vi "Facade.vi"(0 "Data In":T25={"Waveform"={"Type"=enum."Tone", "Tone"={"Frequency (kHz)"=0.0, "Last Freq"=0.0, "Last Phase"=0.0}, "Pulse Train"={"Pulse width (us)"=0.0, "Pulse rate (Hz)"=0.0, "Gap (ms)"=0.0, "Polarity"=enum."POS", "PT State"={"Template"=[], "Nperiod"=0, "Index"=0, "Pulse Rate (Hz)"=0.0, "Phase (cycles)"=0.0, "Noff"=0}, "Asynch"=FALSE}, "Noise"={"InvFilt"=FALSE, "Noise"=[], "CurPt"=0, "Aweight"=FALSE, "Seed"=0, "afile"=path ""}, "File"={"Filename"=path "", "Signal"=[], "Channel"=0, "stream"=FALSE, "offset"=0, "nreps"=0, "loops"=0, "Randomize"=FALSE, "order"=[], "Seed"=0, "Tokens"=0}, "FMSweep"={"Rate (oct/s)"=0.0, "Fmin (Hz)"=0.0, "Fmax (Hz)"=0.0, "Ramp (ms)"=0.0, "Linear"=FALSE}, "Chirp Train"={"Params"={"Fmin (kHz)"=4.0, "Fmax (kHz)"=64.0, "Compensate"=FALSE, "Duration (ms)"=2.0}, "Data"={"WF"=[]}}, "Complex Tone"={"Params"={"F0 (Hz)"=0.0, "Band"={"Flow (Hz)"=0.0, "Fhigh (Hz)"=0.0}, "Phase"=enum."Cosine", "Min F0 (Hz)"=0.0, "Max F0 (Hz)"=0.0, "ContinRandPhase"=FALSE, "Max peak factor"=inf, "Max mod depth"=2.0, "MinHarmNum"=0, "MaxHarmNum"=0, "Level Mode"=enum."per component", "% jitter"=0.0}, "Data"={"Ncomp"=0, "MinHarm"=0, "Phase"=[], "Amplitude"=[], "Npts/frame"=0, "Last F0"=0.0, "Fmin"=0.0, "Fmax"=0.0, "Lslope"=0.0, "randphase"=FALSE, "overall rms"=FALSE, "fmult"=[], "jittered"=FALSE}}, "Moving Ripple"={"Params"={"Fmin"=0.0, "Fmax"=0.0, "Density"=0.0, "Velocity"=0.0, "Depth"=0.0, "Phase"=0.0, "Comp/oct"=0}, "Data"={"Freq"=[], "A"=[], "phase"=[], "Phase"=0.0}}}, "Filter"={"CF (kHz)"=0.0, "BW (kHz)"=0.0, "IIR Filter Cluster"={"filter structure"=enum."IIR 2nd Order", "Reverse Coefficients"=[], "Forward Coefficients"=[]}, "Final Filter State"=[], "Scale Factor"=0.0, "Final Filter State 2"=[], "Quadrature"=FALSE, "Type"=enum."Lowpass"}, "Gate"={"Active"=FALSE, "Delay (ms)"=0.0, "Width (ms)"=50.0, "Ramp (ms)"=5.0}, "Level"={"Level"=0.0, "Units"=enum."dB atten", "Max"=0.0, "Multiplier"=0.0, "Cal File"=path "", "Cal"={"Freq (Hz)"=[], "Mag (dB SPL)"=[], "Phase (deg)"=[]}}} {"Filter"."IIR Filter Cluster"."Forward Coefficients" format="%.4f"; "Filter"."IIR Filter Cluster"."Reverse Coefficients" format="%.4f"}, 2 "Display State In":T23, 3 "Container State":T24) -> (6 "Data Out":T25={"Waveform"={"Type"=enum."Tone", "Tone"={"Frequency (kHz)"=0.0, "Last Freq"=0.0, "Last Phase"=0.0}, "Pulse Train"={"Pulse width (us)"=0.0, "Pulse rate (Hz)"=0.0, "Gap (ms)"=0.0, "Polarity"=enum."POS", "PT State"={"Template"=[], "Nperiod"=0, "Index"=0, "Pulse Rate (Hz)"=0.0, "Phase (cycles)"=0.0, "Noff"=0}, "Asynch"=FALSE}, "Noise"={"InvFilt"=FALSE, "Noise"=[], "CurPt"=0, "Aweight"=FALSE, "Seed"=0, "afile"=path ""}, "File"={"Filename"=path "", "Signal"=[], "Channel"=0, "stream"=FALSE, "offset"=0, "nreps"=0, "loops"=0, "Randomize"=FALSE, "order"=[], "Seed"=0, "Tokens"=0}, "FMSweep"={"Rate (oct/s)"=0.0, "Fmin (Hz)"=0.0, "Fmax (Hz)"=0.0, "Ramp (ms)"=0.0, "Linear"=FALSE}, "Chirp Train"={"Params"={"Fmin (kHz)"=4.0, "Fmax (kHz)"=64.0, "Compensate"=FALSE, "Duration (ms)"=2.0}, "Data"={"WF"=[]}}, "Complex Tone"={"Params"={"F0 (Hz)"=0.0, "Band"={"Flow (Hz)"=0.0, "Fhigh (Hz)"=0.0}, "Phase"=enum."Cosine", "Min F0 (Hz)"=0.0, "Max F0 (Hz)"=0.0, "ContinRandPhase"=FALSE, "Max peak factor"=inf, "Max mod depth"=2.0, "MinHarmNum"=0, "MaxHarmNum"=0, "Level Mode"=enum."per component", "% jitter"=0.0}, "Data"={"Ncomp"=0, "MinHarm"=0, "Phase"=[], "Amplitude"=[], "Npts/frame"=0, "Last F0"=0.0, "Fmin"=0.0, "Fmax"=0.0, "Lslope"=0.0, "randphase"=FALSE, "overall rms"=FALSE, "fmult"=[], "jittered"=FALSE}}, "Moving Ripple"={"Params"={"Fmin"=0.0, "Fmax"=0.0, "Density"=0.0, "Velocity"=0.0, "Depth"=0.0, "Phase"=0.0, "Comp/oct"=0}, "Data"={"Freq"=[], "A"=[], "phase"=[], "Phase"=0.0}}}, "Filter"={"CF (kHz)"=0.0, "BW (kHz)"=0.0, "IIR Filter Cluster"={"filter structure"=enum."IIR 2nd Order", "Reverse Coefficients"=[], "Forward Coefficients"=[]}, "Final Filter State"=[], "Scale Factor"=0.0, "Final Filter State 2"=[], "Quadrature"=FALSE, "Type"=enum."Lowpass"}, "Gate"={"Active"=FALSE, "Delay (ms)"=0.0, "Width (ms)"=50.0, "Ramp (ms)"=5.0}, "Level"={"Level"=0.0, "Units"=enum."dB atten", "Max"=0.0, "Multiplier"=0.0, "Cal File"=path "", "Cal"={"Freq (Hz)"=[], "Mag (dB SPL)"=[], "Phase (deg)"=[]}}} {"Filter"."IIR Filter Cluster"."Forward Coefficients" format="%.4f"; "Filter"."IIR Filter Cluster"."Reverse Coefficients" format="%.4f"}, 7 "Display State Out":T23, 8 "Action":T22)   [LabVIEW 2020, in "Stimulus Channel.xctl"]
uses:
  Stimulus Channel.xctl
  Stimulus Channel Data.ctl
  Waveform XCtl/Waveform Data.ctl
  Waveform XCtl/Waveform Enum.ctl
  Waveform VIs/Tone VIs/Tone Params.ctl
  Waveform VIs/Pulse Train VIs/Pulse Train Params.ctl
  Waveform VIs/Pulse Train VIs/Pulse Polarity.ctl
  Waveform VIs/Pulse Train VIs/PT-Continuous State.ctl
  Waveform VIs/Noise VIs/Noise Params.ctl
  Waveform VIs/File VIs/StimFile-Params.ctl
  Waveform VIs/FM Sweep VIs/FM Sweep Params.ctl
  Waveform VIs/Chirp Train VIs/Chirp Train.ctl
  Waveform VIs/Chirp Train VIs/Chirp Train Params.ctl
  Waveform VIs/Complex Tone VIs/CT-Params.ctl
  Waveform VIs/Complex Tone VIs/CT-Phase Enum.ctl
  Waveform VIs/Complex Tone VIs/CT-Runtime Data.ctl
  Waveform VIs/Moving Ripple VIs/Moving Ripple.ctl
  Waveform VIs/Moving Ripple VIs/Moving Ripple.Params.ctl
  Waveform VIs/Moving Ripple VIs/Moving Ripple.Data.ctl
  Filter XCtl/Filter Data.ctl
  Gate XCtl/Gate Data.ctl
  Level XCtl/Level Data.ctl
  Level XCtl/Level Units.ctl
  <vilib>/_xctls/Container State.ctl
  State.ctl
  <vilib>/_xctls/Action.ctl
  Filter XCtl/Filter XCtl.xctl
  Level XCtl/Level XCtl.xctl
  Gate XCtl/Gate Control.xctl
  Waveform XCtl/Waveform XCtl.xctl
  <vilib>/_xctls/XControlSupport.lvlib
panel:
  in  "Waveform":T17(xcontrol)
  in  "Gate":T18(xcontrol)
  in  "Level":T20(xcontrol)
  in  "Filter":T21(xcontrol)
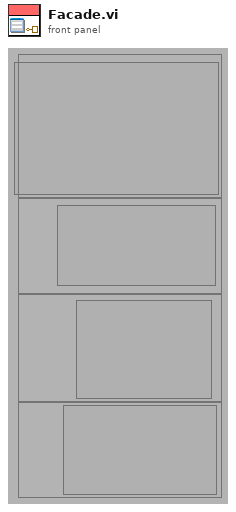
[diagram p1: front panel]
types:
  T1 = typedef "Waveform Enum.ctl" = enum16{"OFF", "Tone", "Noise", "Pulse Train", "File", "FM Sweep", "Chirp Train", "Complex Tone", "FM Tone", "Moving Ripple"}
  T2 = typedef "Tone Params.ctl" = cluster{"Frequency (kHz)":dbl, "Last Freq":dbl, "Last Phase":dbl}
  T3 = typedef "Pulse Train Params.ctl" = cluster{"Pulse width (us)":dbl, "Pulse rate (Hz)":dbl, "Gap (ms)":dbl, "Polarity":T4, "PT State":T5, "Asynch":bool}
  T4 = typedef "Pulse Polarity.ctl" = enum16{"POS", "NEG", "POS-NEG", "NEG-POS"}
  T5 = typedef "PT-Continuous State.ctl" = cluster{"Template":dbl[], "Nperiod":i32, "Index":i32, "Pulse Rate (Hz)":dbl, "Phase (cycles)":dbl, "Noff":i32}
  T6 = typedef "Noise Params.ctl" = cluster{"InvFilt":bool, "Noise":dbl[], "CurPt":i32, "Aweight":bool, "Seed":i32, "afile":path}
  T7 = typedef "StimFile-Params.ctl" = cluster{"Filename":path, "Signal":dbl[], "Channel":i32, "stream":bool, "offset":i32, "nreps":i32, "loops":i32, "Randomize":bool, "order":i32[], "Seed":i32, "Tokens":i32}
  T8 = typedef "FM Sweep Params.ctl" = cluster{"Rate (oct/s)":dbl, "Fmin (Hz)":dbl, "Fmax (Hz)":dbl, "Ramp (ms)":dbl, "Linear":bool}
  T9 = typedef "Chirp Train.ctl" = cluster{"Params":T10, "Data":cluster{"WF":dbl[]}}
  T10 = typedef "Chirp Train Params.ctl" = cluster{"Fmin (kHz)":dbl, "Fmax (kHz)":dbl, "Compensate":bool, "Duration (ms)":dbl}
  T11 = typedef "CT-Params.ctl" = cluster{"F0 (Hz)":dbl, "Band":cluster{"Flow (Hz)":dbl, "Fhigh (Hz)":dbl}, "Phase":T12, "Min F0 (Hz)":dbl, "Max F0 (Hz)":dbl, "ContinRandPhase":bool, "Max peak factor":dbl, "Max mod depth":dbl, "MinHarmNum":i32, "MaxHarmNum":i32, "Level Mode":enum16{"per component", "overall rms"}, "% jitter":dbl}
  T12 = typedef "CT-Phase Enum.ctl" = enum16{"Cosine", "Random", "Alternating"}
  T13 = typedef "CT-Runtime Data.ctl" = cluster{"Ncomp":i32, "MinHarm":i32, "Phase":dbl[], "Amplitude":dbl[], "Npts/frame":i32, "Last F0":dbl, "Fmin":dbl, "Fmax":dbl, "Lslope":dbl, "randphase":bool, "overall rms":bool, "fmult":dbl[], "jittered":bool}
  T14 = typedef "Moving Ripple.ctl" = cluster{"Params":T15, "Data":T16}
  T15 = typedef "Moving Ripple.Params.ctl" = cluster{"Fmin":dbl, "Fmax":dbl, "Density":dbl, "Velocity":dbl, "Depth":dbl, "Phase":dbl, "Comp/oct":i32}
  T16 = typedef "Moving Ripple.Data.ctl" = cluster{"Freq":dbl[], "A":dbl[], "phase":dbl[], "Phase":dbl}
  T17 = cluster{"Type":T1, "Tone":T2, "Pulse Train":T3, "Noise":T6, "File":T7, "FMSweep":T8, "Chirp Train":T9, "Complex Tone":cluster{"Params":T11, "Data":T13}, "Moving Ripple":T14}
  T18 = cluster{"Active":bool, "Delay (ms)":dbl, "Width (ms)":dbl, "Ramp (ms)":dbl}
  T19 = typedef "Level Units.ctl" = enum16{"dB atten", "dB SPL", "dB re 1 Vrms", "dB V/Hz½", "mW", "dB HL", "Volts", "dB mW"}
  T20 = cluster{"Level":dbl, "Units":T19, "Max":dbl, "Multiplier":dbl, "Cal File":path, "Cal":cluster{"Freq (Hz)":dbl[], "Mag (dB SPL)":dbl[], "Phase (deg)":dbl[]}}
  T21 = cluster{"CF (kHz)":dbl, "BW (kHz)":dbl, "IIR Filter Cluster":cluster{"filter structure":enum32{"IIR 2nd Order", "IIR 4th Order"}, "Reverse Coefficients":dbl[], "Forward Coefficients":dbl[]}, "Final Filter State":dbl[], "Scale Factor":dbl, "Final Filter State 2":dbl[], "Quadrature":bool, "Type":enum16{"Lowpass", "Highpass", "Bandpass", "Bandstop", "OFF"}}
  T22 = typedef "XControlSupport.lvlib/Action.ctl" = cluster{"Data Changed?":bool, "State Changed?":bool, "Action Name":string}
  T23 = typedef "Stimulus Channel.xctl/State.ctl" = cluster{"Update":bool}
  T24 = typedef "XControlSupport.lvlib/Container State.ctl" = cluster{"Indicator?":bool, "Run Mode?":bool, " Refnum":refnum<vi>}
  T25 = typedef "Stimulus Channel.xctl/Stimulus Channel Data.ctl" = cluster{"Waveform":T26, "Filter":T27, "Gate":T28, "Level":T29}
  T26 = typedef "Waveform XCtl.xctl/Waveform Data.ctl" = cluster{"Type":T1, "Tone":T2, "Pulse Train":T3, "Noise":T6, "File":T7, "FMSweep":T8, "Chirp Train":T9, "Complex Tone":cluster{"Params":T11, "Data":T13}, "Moving Ripple":T14}
  T27 = typedef "Filter XCtl.xctl/Filter Data.ctl" = cluster{"CF (kHz)":dbl, "BW (kHz)":dbl, "IIR Filter Cluster":cluster{"filter structure":enum32{"IIR 2nd Order", "IIR 4th Order"}, "Reverse Coefficients":dbl[], "Forward Coefficients":dbl[]}, "Final Filter State":dbl[], "Scale Factor":dbl, "Final Filter State 2":dbl[], "Quadrature":bool, "Type":enum16{"Lowpass", "Highpass", "Bandpass", "Bandstop", "OFF"}}
  T28 = typedef "Gate Control.xctl/Gate Data.ctl" = cluster{"Active":bool, "Delay (ms)":dbl, "Width (ms)":dbl, "Ramp (ms)":dbl}
  T29 = typedef "Level XCtl.xctl/Level Data.ctl" = cluster{"Level":dbl, "Units":T19, "Max":dbl, "Multiplier":dbl, "Cal File":path, "Cal":cluster{"Freq (Hz)":dbl[], "Mag (dB SPL)":dbl[], "Phase (deg)":dbl[]}}
  T30 = enum8{"Enabled", "Disabled", "Disabled and Grayed Out"}
  T31 = enum16{"Lowpass", "Highpass", "Bandpass", "Bandstop", "OFF"}
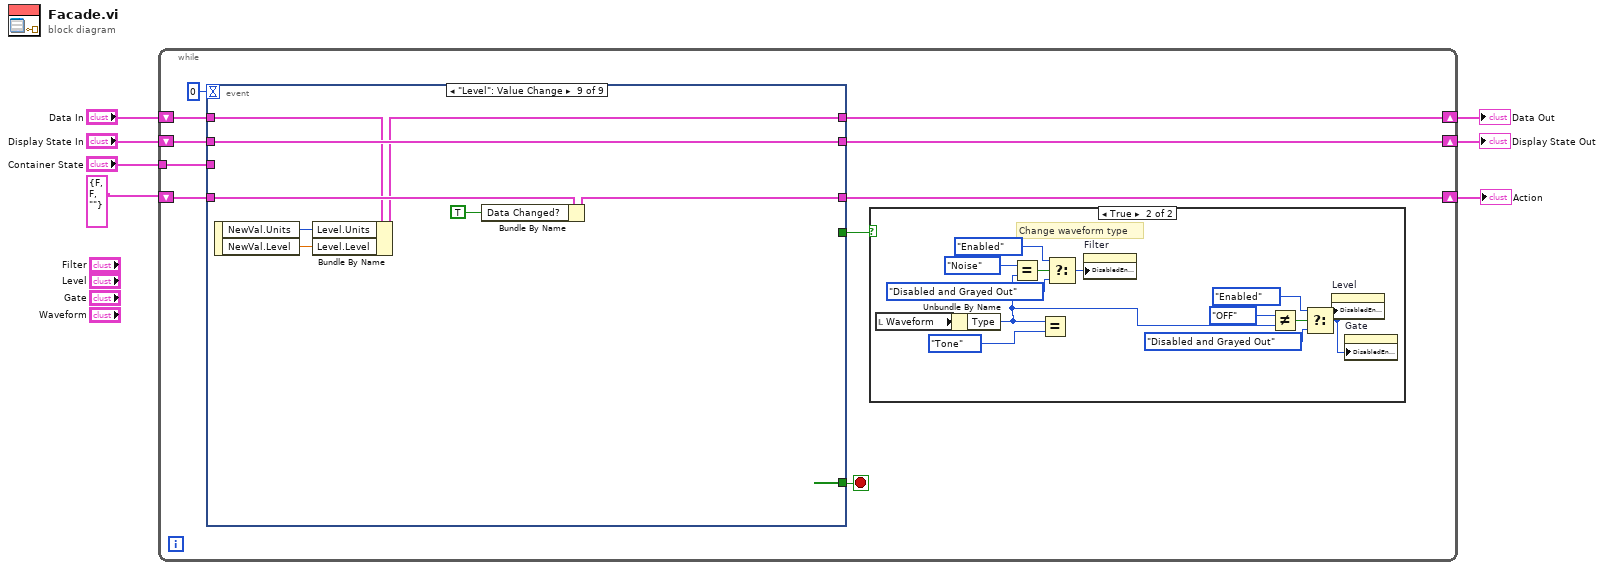
[diagram p0: block diagram]
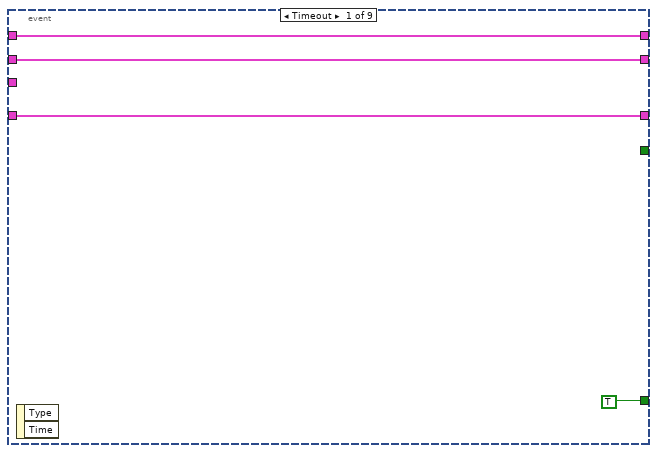
[diagram p3: hidden frame]
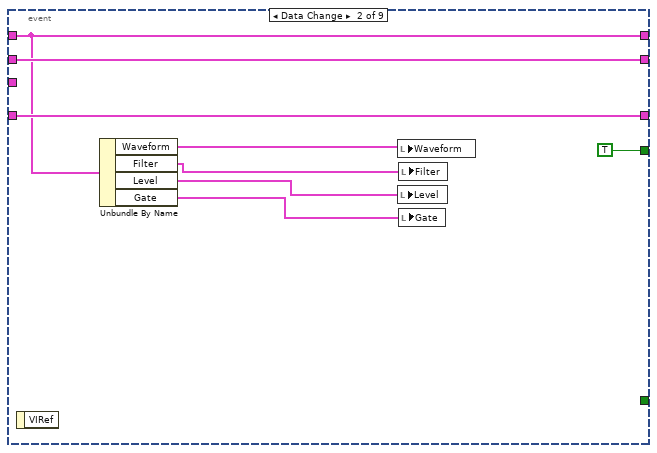
[diagram p4: hidden frame]
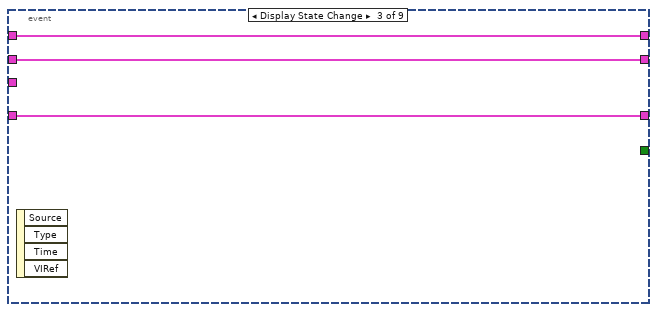
[diagram p5: hidden frame]
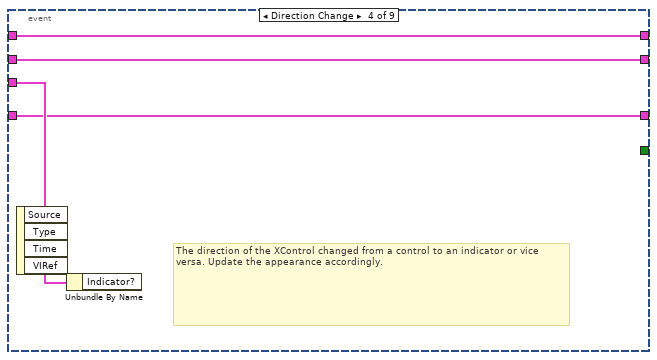
[diagram p6: hidden frame]
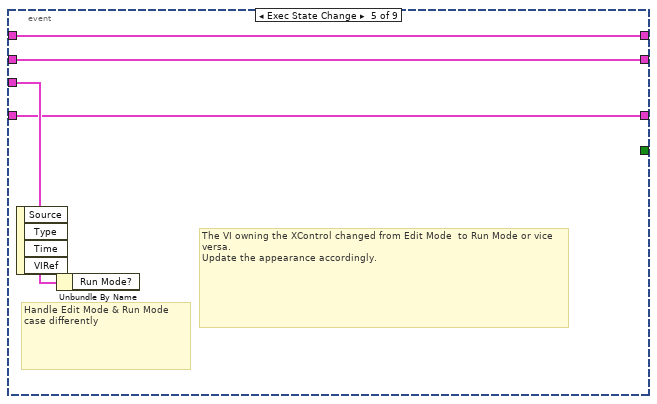
[diagram p7: hidden frame]
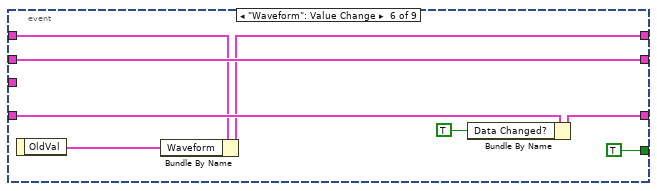
[diagram p8: hidden frame]
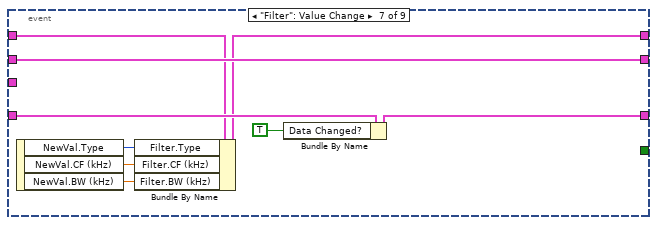
[diagram p9: hidden frame]
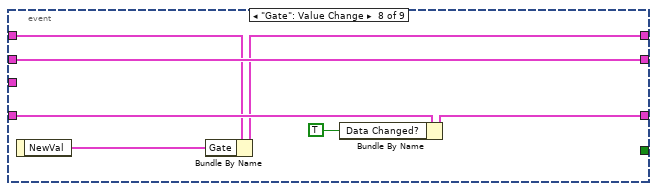
[diagram p10: hidden frame]
diagram:
  n1 = while {
    shift-right: [w16] -> w4
    shift-left: "Display State In" -> [w17]
    tunnel: "Container State" -> [w13]
    shift-right: [w11] -> w7
    shift-left: "Data In" -> [w12]
    shift-right: [w9] -> w2
    shift-left: T22 {"Data Changed?"=FALSE, "State Changed?"=FALSE, "Action Name"=""} ("Action") -> [w10]
    stop <- w15 stop-if-true
    n2 = event shown="[8] \"Level\": Value Change" {
      selector: _ -> [_ _ _ _ _ _ _ _ _]
      dyn-events: _ -> [_ _ _ _ _ _ _ _ _]
      timeout: 0 -> [_ _ _ _ _ _ _ _ _]
      tunnel: w17 -> [w32 w42 w44 w48 w52 w57 w67 w74 w82]
      tunnel: [w32 w42 w44 w48 w52 w57 w67 w74 w82] -> w16
      tunnel: [TRUE _ _ _ _ _ _ _ _] -> w15
      tunnel: w13 -> [_ _ _ w49 w53 _ _ _ _]
      tunnel: w12 -> [w31 w40 w45 w47 w51 w56 w66 w73 w81]
      tunnel: [w31 w40 w45 w47 w51 w55 w65 w72 w80] -> w11
      tunnel: [w33 w41 w43 w46 w50 w58 w68 w75 w83] -> w9
      tunnel: w10 -> [w33 w41 w43 w46 w50 w60 w70 w77 w85]
      tunnel: [_ TRUE _ _ _ TRUE _ _ _] -> w8
      event Timeout {
        n3 = event-data() -> ()  [unwired: 1 in, 2 out]
      }
      event Data Change {
        n4 = event-data() -> ()  [unwired: 1 in, 1 out]
        n5 = Unbundle By Name(w40) -> ("Waveform"=w38:T26, "Filter"=w36:T27, "Level"=w35:T29, "Gate"=w37:T28)
        n6 = local write "Waveform"(w38) -> ()
        n7 = local write "Level"(w35) -> ()
        n8 = local write "Filter"(w36) -> ()
        n9 = local write "Gate"(w37) -> ()
      }
      event Display State Change {
        n10 = event-data() -> ()  [unwired: 1 in, 4 out]
      }
      event Direction Change {
        # "The direction of the XControl changed from a control to an indicator or vice versa. Update the appearance accordingly."
        n11 = event-data() -> ()  [unwired: 1 in, 4 out]
        n12 = Unbundle By Name(w49) -> ()  [unwired: 1 out]
      }
      event Exec State Change {
        # "The VI owning the XControl changed from Edit Mode  to Run Mode or vice versa.\nUpdate the appearance accordingly."
        # "Handle Edit Mode & Run Mode\ncase differently"
        n13 = event-data() -> ()  [unwired: 1 in, 4 out]
        n14 = Unbundle By Name(w53) -> ()  [unwired: 1 out]
      }
      event "Waveform": Value Change {
        n15 = event-data() -> ("OldVal"=w54:T17)  [unwired: 1 in]
        n16 = Bundle By Name(cluster=w56, "Waveform"=w54) -> (w55:T25)
        n17 = Bundle By Name(cluster=w60, "Data Changed?"=TRUE) -> (w58:T22)
      }
      event "Filter": Value Change {
        n18 = event-data() -> ("NewVal.Type"=w64:T31, "NewVal.CF (kHz)"=w63:dbl, "NewVal.BW (kHz)"=w62:dbl)  [unwired: 1 in]
        n19 = Bundle By Name(cluster=w66, "Filter.Type"=w64, "Filter.CF (kHz)"=w63, "Filter.BW (kHz)"=w62) -> (w65:T25)
        n20 = Bundle By Name(cluster=w70, "Data Changed?"=TRUE) -> (w68:T22)
      }
      event "Gate": Value Change {
        n21 = event-data() -> ("NewVal"=w71:T18)  [unwired: 1 in]
        n22 = Bundle By Name(cluster=w73, "Gate"=w71) -> (w72:T25)
        n23 = Bundle By Name(cluster=w77, "Data Changed?"=TRUE) -> (w75:T22)
      }
      event "Level": Value Change {
        n24 = event-data() -> ("NewVal.Units"=w79:T19, "NewVal.Level"=w78:dbl)  [unwired: 1 in]
        n25 = Bundle By Name(cluster=w81, "Level.Units"=w79, "Level.Level"=w78) -> (w80:T25)
        n26 = Bundle By Name(cluster=w85, "Data Changed?"=TRUE) -> (w83:T22)
      }
    }
    n27 = case shown="True" w8 {
      frame False {
      }
      frame True {
        # "Change waveform type"
        n28 = local read "Waveform"() -> (w20:T17)
        n29 = Unbundle By Name(w20) -> ("Type"=w19:T1)
        n30 = Equal?(x=enum16{"OFF", "Tone", "Noise"}."Noise", y=w19) -> (x = y?=w30:bool)
        n31 = Equal?(x=w19, y=enum16{"OFF", "Tone", "Noise"}."Tone") -> ()  [unwired: 1 out]
        n32 = Select(t=T30."Enabled" ("Disabled"), s=w30, f=T30."Disabled and Grayed Out" ("Disabled")) -> (s? t:f=w27:T30)
        n33 = property on="Filter" class="Filter XCtl (strict)"("DisabledEnum"=w27) -> ()  [unwired: 2 in, 2 out]
        n34 = Not Equal?(x=enum16{"OFF", "Tone", "Noise"}."OFF", y=w19) -> (x != y?=w25:bool)
        n35 = Select(t=T30."Enabled" ("Disabled"), s=w25, f=T30."Disabled and Grayed Out" ("Disabled")) -> (s? t:f=w18:T30)
        n36 = property on="Level" class="Level XCtl (strict)"("DisabledEnum"=w18) -> ()  [unwired: 2 in, 2 out]
        n37 = property on="Gate" class="Gate Control (strict)"("DisabledEnum"=w18) -> ()  [unwired: 2 in, 2 out]
      }
    }
  }
  "Display State Out" <- w4
  "Data Out" <- w7
  "Action" <- w2
